vi "Close.vi"(8 "error in (no error)":errorcluster, 11 "Dynamic Combobox in":refnum<class "Dynamic Combobox.lvclass">) -> (0 "error out":errorcluster)   [LabVIEW 2020, in "Dynamic Combobox.lvlib" / "Dynamic Combobox.lvclass"]
uses:
  Dynamic Combobox.lvclass
  Dynamic Combobox.lvclass/Dynamic Combobox.ctl
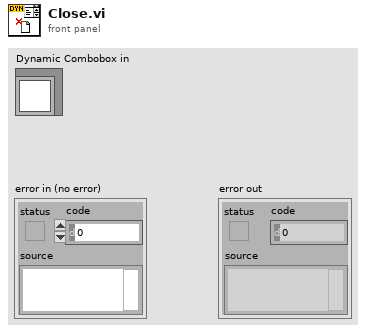
[diagram p1: front panel]
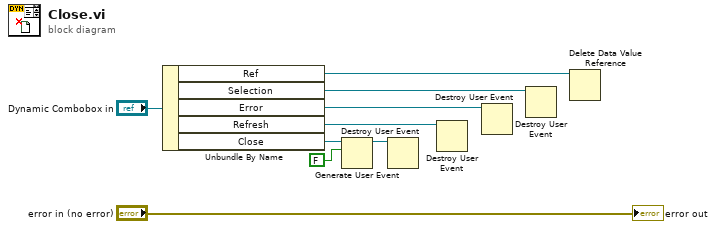
[diagram p0: block diagram]
diagram:
  n1 = Unbundle By Name("Dynamic Combobox in") -> ("Ref"=w1:refnum<data-value>, "Selection"=w2:refnum<user-event>, "Error"=w3:refnum<user-event>, "Refresh"=w4:refnum<user-event>, "Close"=w7:refnum<user-event>)
  n2 = Generate User Event(user event=w7, event data cluster=FALSE ("event data")) -> (user event out=w5:refnum<user-event>)  [unwired: 2 in, 1 out]
  n3 = Destroy User Event(user event=w5) -> ()  [unwired: 1 in, 1 out]
  n4 = Destroy User Event(user event=w4) -> ()  [unwired: 1 in, 1 out]
  n5 = Destroy User Event(user event=w3) -> ()  [unwired: 1 in, 1 out]
  n6 = Destroy User Event(user event=w2) -> ()  [unwired: 1 in, 1 out]
  n7 = Delete Data Value Reference(data value reference=w1) -> ()  [unwired: 1 in, 2 out]
  "error out" <- "error in (no error)"
